vi "Configure Pulse Waveform_Width.vi"(4 "Width(s)":dbl=50.0, 5 "Trailing Edge Time (5.0E-8)":dbl=5e-08 format="%#.6g", 6 "Delay (0 s)":dbl, 7 "Leading Edge Time (5.0E-8)":dbl=5e-08 format="%#.6g", 8 "error in (no error)":errorcluster, 9 "Period(s)":dbl=50.0, 10 "Channel (0: Channel 1)":u16(ring) items=["Channel 1", "Channel 2"], 11 "VISA resource name":refnum<visa-resource-name>) -> (0 "error out":errorcluster, 3 "VISA resource name out":refnum<visa-resource-name>)   [LabVIEW 2019]
doc: "Configures parameters for pulse waveforms which include channel, leading edge time, trailing edge time, duty cycle, and delay."
uses:
  <userlib>/Tektronix AFG 3000 Series/Tektronix AFG 3000 Series.lvlib
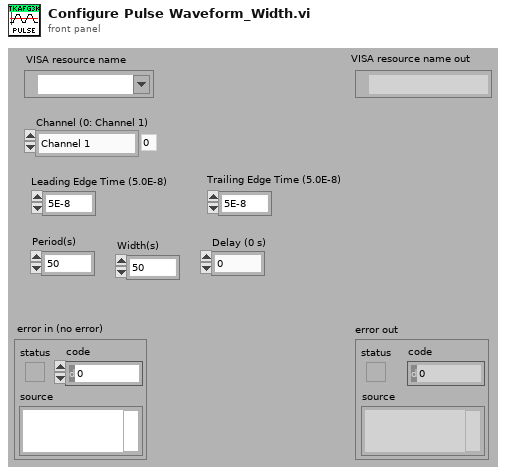
[diagram p1: front panel]
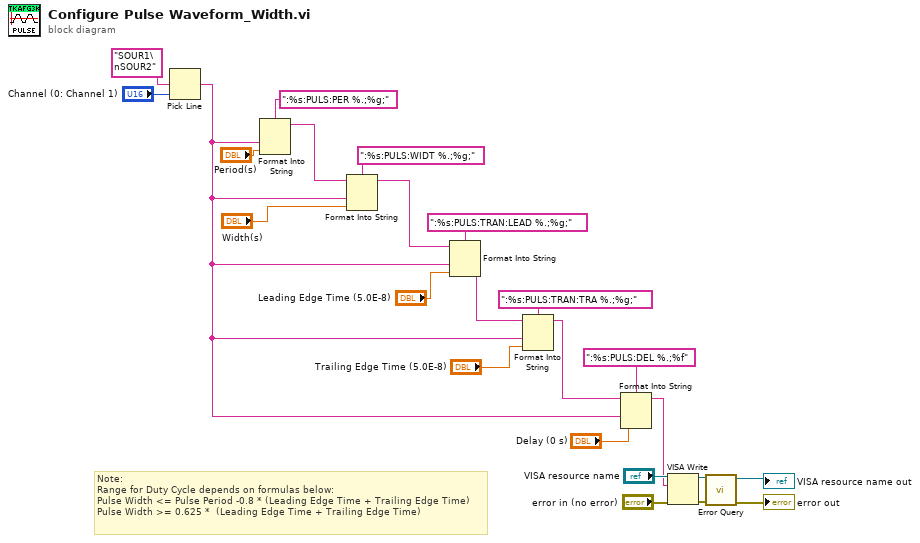
[diagram p0: block diagram]
diagram:
  # "Note:\nRange for Duty Cycle depends on formulas below:\nPulse Width <= Pulse Period -0.8 * (Leading Edge Time + Trailing Edge Time)\nPulse Width >= 0.625 *  (Leading Edge Time + Trailing Edge Time)"
  n1 = Pick Line(multi-line string="SOUR1\nSOUR2" ("string (\"\")"), line index="Channel (0: Channel 1)") -> (output string=w1:string)  [unwired: 1 in]
  n2 = Format Into String(format string=":%s:PULS:PER %.;%g;", w1, "Period(s)") -> (resulting string=w4:string)  [unwired: 2 in, 1 out]
  n3 = Format Into String(format string=":%s:PULS:WIDT %.;%g;", initial string=w4, w1, "Width(s)") -> (resulting string=w3:string)  [unwired: 1 in, 1 out]
  n4 = Format Into String(format string=":%s:PULS:TRAN:LEAD %.;%g;", initial string=w3, w1, "Leading Edge Time (5.0E-8)") -> (resulting string=w17:string)  [unwired: 1 in, 1 out]
  n5 = Format Into String(format string=":%s:PULS:TRAN:TRA %.;%g;", initial string=w17, w1, "Trailing Edge Time (5.0E-8)") -> (resulting string=w8:string)  [unwired: 1 in, 1 out]
  n6 = Format Into String(format string=":%s:PULS:DEL %.;%f" ("string"), initial string=w8, w1, "Delay (0 s)") -> (resulting string=w6:string)  [unwired: 1 in, 1 out]
  n7 = VISA Write(VISA resource name="VISA resource name", write buffer=w6, error in (no error)="error in (no error)") -> (VISA resource name out=w22:refnum<visa-resource-name>, error out=w21:errorcluster)  [unwired: 1 out]
  n8 = call <userlib>:"Error Query.vi"("error in (no error)"=w21, "VISA resource name"=w22) -> ("error out"=→"error out":errorcluster, "VISA resource name out"=→"VISA resource name out":refnum<visa-resource-name>)  [unwired: 6 in, 2 out]
